vi "Get Part Names.vi"(8 "error in":errorcluster, 9 "Read Edit Tolerance \nOverride JSON":path=path "C:/Users/raakeshs/Desktop/GTRON/JSONs/DeafultJSON_Final.json", 10 "Part Name":string, 11 "Algo Override\nJSON Variant in":variant) -> (0 "error out":errorcluster, 3 "Measurement Names":string[](array[string]))   [LabVIEW 2015, in "ZenGage v3.0 UI.lvclass"]
uses:
  ZenGage v3.0 UI.lvclass
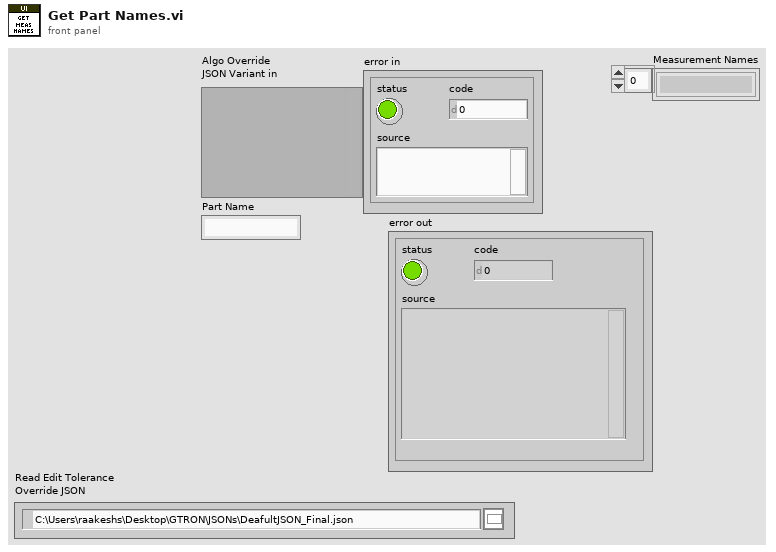
[diagram p1: front panel]
types:
  T1 = typedef "ZenGage v3.0 UI.lvclass/Algo(Override).ctl" = cluster{"AlgoParameters":cluster{"PartsList":cluster{"Name":string, "Measurements":cluster{"RackID":i32, "MeasurementId":i32, "Name":string, "AlgoName":string, "MeasurementEnable":bool, "Calibration Coefficients":cluster{"Linearity Correction":dbl, "Bias Correction":dbl}, "SpecValues":cluster{"LCL":dbl, "UCL":dbl, "LSL":dbl, "USL":dbl, "NominalValue":dbl}}[]}[]}}
  T2 = cluster{"Name":string, "Measurements":cluster{"RackID":i32, "MeasurementId":i32, "Name":string, "AlgoName":string, "MeasurementEnable":bool, "Calibration Coefficients":cluster{"Linearity Correction":dbl, "Bias Correction":dbl}, "SpecValues":cluster{"LCL":dbl, "UCL":dbl, "LSL":dbl, "USL":dbl, "NominalValue":dbl}}[]}[]
  T3 = cluster{"Name":string, "Measurements":cluster{"RackID":i32, "MeasurementId":i32, "Name":string, "AlgoName":string, "MeasurementEnable":bool, "Calibration Coefficients":cluster{"Linearity Correction":dbl, "Bias Correction":dbl}, "SpecValues":cluster{"LCL":dbl, "UCL":dbl, "LSL":dbl, "USL":dbl, "NominalValue":dbl}}[]}
  T4 = cluster{"RackID":i32, "MeasurementId":i32, "Name":string, "AlgoName":string, "MeasurementEnable":bool, "Calibration Coefficients":cluster{"Linearity Correction":dbl, "Bias Correction":dbl}, "SpecValues":cluster{"LCL":dbl, "UCL":dbl, "LSL":dbl, "USL":dbl, "NominalValue":dbl}}[]
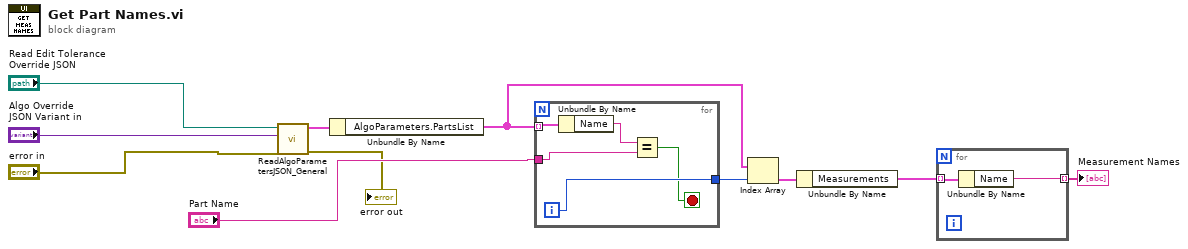
[diagram p0: block diagram]
diagram:
  n1 = call "ReadAlgoParametersJSON_General.vi"("error in"="error in", "Algo Override\nJSON Variant in"="Algo Override\nJSON Variant in", "Read Edit Tolerance \nOverride JSON"="Read Edit Tolerance \nOverride JSON") -> ("error out"=→"error out":errorcluster, "AlgoParameters (Override) Cluster out"=w11:T1)  [unwired: 6 in, 1 out]
  n2 = Unbundle By Name(w11) -> ("AlgoParameters.PartsList"=w8:T2)
  n3 = for {
    tunnel: "Part Name" -> [w14]
    tunnel: w8 -> [w16] mode=indexing
    tunnel: [w13] -> w9
    i -> [w13]
    stop <- w12 stop-if-true
    n4 = Unbundle By Name(w16) -> ("Name"=w15:string)
    n5 = Equal?(x=w15, y=w14) -> (x = y?=w12:bool)
  }
  n6 = Index Array(array=w8, index=w9) -> (element=w7:T3)
  n7 = Unbundle By Name(w7) -> ("Measurements"=w6:T4)
  n8 = for {
    tunnel: w6 -> [w18] mode=indexing
    tunnel: [w17] -> w5 mode=indexing
    n9 = Unbundle By Name(w18) -> ("Name"=w17:string)
  }
  "Measurement Names" <- w5
